vi "New Measurement Cluster Constant.vi"(11 "Bitfile name":string) -> (3 "Measurement":T1={"Name"="", "Bitfile name"="", "Window"="", "Polarity"=enum."Active high"})   [LabVIEW 2019, in "Engine Simulation Toolkit System Explorer.lvlib"]
uses:
  Engine Simulation Toolkit System Explorer.lvlib
  Event Timing Measurement.ctl
  Polarity.ctl
  Shared/Constants and GUIDs.vi
  Shared/Engine Simulation Toolkit Shared.lvlib
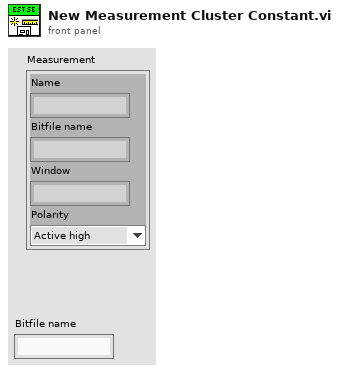
[diagram p1: front panel]
types:
  T1 = typedef "Engine Simulation Toolkit System Explorer.lvlib/Event Timing Measurement.ctl" = cluster{"Name":string, "Bitfile name":string, "Window":string, "Polarity":T2}
  T2 = typedef "Engine Simulation Toolkit System Explorer.lvlib/Polarity.ctl" = enum16{"Active low", "Active high"}
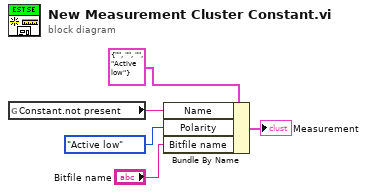
[diagram p0: block diagram]
diagram:
  n1 = global read "Constants and GUIDs.vi" "Constant.not present"() -> (w3:string)
  n2 = Bundle By Name(cluster=T1 {"Name"="", "Bitfile name"="", "Window"="", "Polarity"=enum."Active low"} ("Window"), "Name"=w3, "Polarity"=Polarity."Active low", "Bitfile name"="Bitfile name") -> (→"Measurement":T1)
